vi "Step 4 - Model and Simulate FXP Decimation (NStageMRate).vi"() -> ()   [LabVIEW 2023]
doc: "Demonstrates how to use the DFD FXP NStage MRate Modeling VI to model a 3-stage fixed-point filter, the DFD FXP NStage MRate Simulation VI to simulate the filtering process, and the DFD NStage MRate Filtering VI to get the reference floating-point filtering results.\n\nThis example uses the DFD FXP NStage MRate Modeling VI to create a model of the fixed-point multistage decimation filter. The example then uses the DFD FXP NStage MRate Simulation VI to apply the fixed-point decimation filter model to a signal from the Uniform White Noise VI and simulates the filtering result. To verify the simulation, this example also uses the DFD NStage MRate Filtering VI to filter the same signal that the Uniform White Noise VI generates with the original reference floating-point multistage decimation filter and finally uses the MSE VI to compute the mean squared error (MSE) of the two filtered signals.\n\nAfter you run the VI, compare the signal from the reference floating-point multistage decimation filter and the signal from the fixed-point multistage decimation filter model. The ideal result is that the two signals overlap each other."
uses:
  <vilib>/addons/Digital Filter Design/FXPMRateSim.llb/DFD FXP NStage MRate Simulation (DBL).vi
  <vilib>/addons/Digital Filter Design/Multirate.llb/DFD NStage MRate Filtering (Array).vi
  <vilib>/addons/Digital Filter Design/NI_DigFilterLicensed.lvlib
  <vilib>/Analysis/NI_AALPro.lvlib
  <vilib>/Analysis/NI_AALBase.lvlib
panel:
  out "MSE":dbl format="%.3g"
  out "Filtered Signals":dbl[][](graph)
  # "Select Help>>Show Context Help and move the cursor over the VI icon for more information."
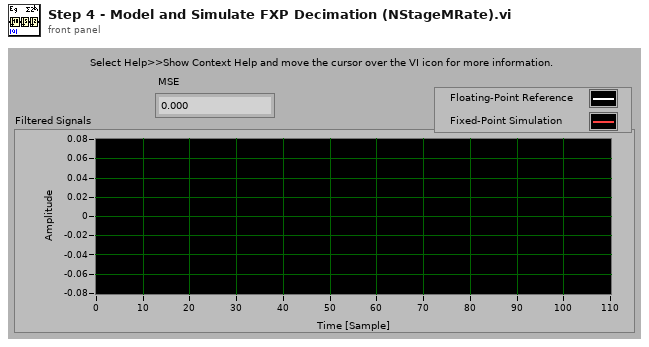
[diagram p1: front panel]
types:
  T1 = typedef "NI_DigFilterLicensed.lvlib/DFD Multirate Filter Obj.ctl" = cluster{"mMRate_Structure":enum16{"CIC", "FIR", "IIR", "Lattice"}, "mMRate_Mode":T2, "mMRate_Factor":i32, "mMRate_FIRParams":cluster{"mMRate_FIR_H":dbl[], "mMRate_FIR_IsNyquist?":bool, "mMRate_FIR_IsSymmetric?":bool}, "mMRate_CICParams":cluster{"mMRate_CIC_#Stage":i32, "mMRate_CIC_Lag":i32, "mMRate_CIC_Type":enum16{"Lowpass", "Highpass"}}, "mMRate_Order":i32, "mMRate_Version":string, "mMRate_Comments":string, "mMRate_RationalFactor":cluster{"mMRate_L":i32, "mMRate_M":i32}, "mMRate_Fs":dbl, "mMRate_Quantized?":bool, "mMRate_QFilterGain":dbl, "mMRate_CoefWl":i16, "mMRate_Scaling":cluster{"mMRate_ScaleByPowerOf2?":bool, "mMRate_ScaleType":T3}, "mMRate_InputWl":i16, "mMRate_OutputWl":i16, "mMRate_OutputMode":T4, "mMRate_MultMode":T5, "mMRate_BitPruning":bool, "mMRate_GainWl":i16, "mMRate_OutputFwl":i16, "mMRate_SumIwl":i16, "mMRate_InputIwl ":i16, "mMRate_SumWl":i16, "mMRate_CoefIwl":i16}
  T2 = typedef "NI_DigFilterLicensed.lvlib/DFD Multirate Mode.ctl" = i16
  T3 = typedef "NI_DigFilterLicensed.lvlib/DFD Coef Norm Type.ctl" = enum16{"No Norm", "Time Domain 1-Norm", "Time Domain 2-Norm", "Time Domain Inf-Norm"}
  T4 = typedef "NI_DigFilterLicensed.lvlib/DFD Round-off Mode.ctl" = enum16{"Nearest", "Truncation"}
  T5 = typedef "NI_DigFilterLicensed.lvlib/DFD FXP MRate Multiply Mode.ctl" = enum16{"Truncated", "Full"}
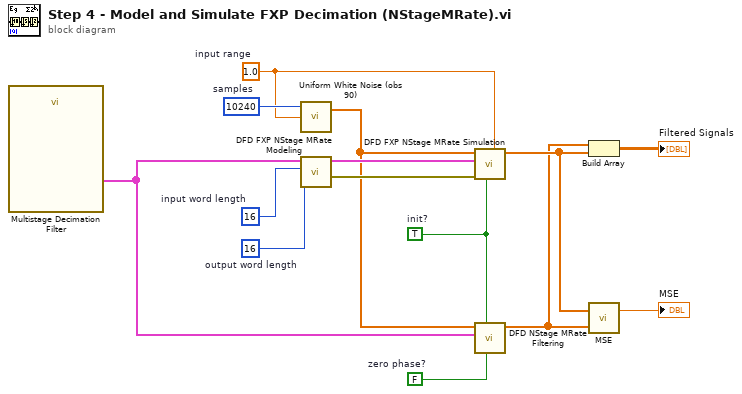
[diagram p0: block diagram]
diagram:
  w2 = i16 16  # output word length
  w3 = i16 16  # input word length
  w6 = 1.0  # input range
  w12 = FALSE  # zero phase?
  w5 = TRUE  # init?
  w14 = 10240  # samples
  n1 = call "Multistage Decimation Filter"() -> ("multirate filters out"=w1:T1[])  [unwired: 11 out]
  n2 = call <vilib>:"Uniform White Noise (obs 90).vi"("amplitude"=w6, "samples"=w14) -> ("uniform white noise"=w4:dbl[])  [unwired: 1 in, 1 out]
  n3 = call <vilib>:"DFD FXP NStage MRate Modeling.vi"("output word length"=w2, "input word length"=w3, "multirate filters in"=w1) -> ("error out"=w7:errorcluster, "multirate filters out"=w13:T1[])  [unwired: 5 in, 2 out]
  n4 = call-poly <vilib>:"DFD FXP NStage MRate Simulation.vi"("input range"=w6, "init? (T)"=w5, "error in (no error)"=w7, "multirate filters"=w13, "signal in"=w4) -> ("DBL signal out"=w9:dbl[])  [unwired: 6 out]
  n5 = call-poly <vilib>:"DFD NStage MRate Filtering.vi"("zero phase? (T)"=w12, "init? (F)"=w5, "multirate filters"=w1, "signal in"=w4) -> ("signal out"=w8:dbl[])  [unwired: 1 in, 6 out]
  n6 = Build Array(w8, w9) -> (→"Filtered Signals":dbl[][])
  n7 = call <vilib>:"MSE.vi"("X Values"=w8, "Y Values"=w9) -> ("mse"=→"MSE":dbl)  [unwired: 1 out]
